vi "Set_up_measurement.vi"(4 "error in (no error)":errorcluster, 5 "VISA resource name":refnum<visa-resource-name>) -> (1 "error out":errorcluster, 2 "VISA resource name out":refnum<visa-resource-name>)   [LabVIEW 2021]
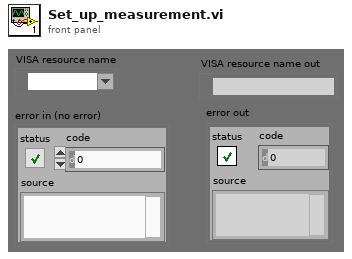
[diagram p1: front panel]
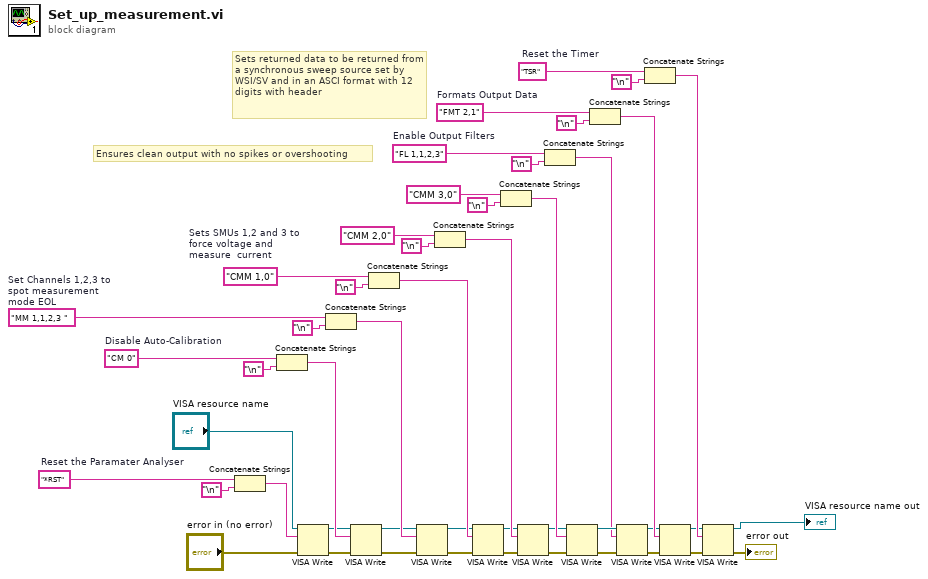
[diagram p0: block diagram]
diagram:
  w9 = "CM 0"  # Disable Auto-Calibration
  w12 = "*RST"  # Reset the Paramater Analyser
  w21 = "FMT 2,1"  # Formats Output Data
  w24 = "TSR"  # Reset the Timer
  w27 = "FL 1,1,2,3"  # Enable Output Filters
  w43 = "CMM 1,0"  # Sets SMUs 1,2 and 3 to force voltage and measure  current
  w47 = "MM 1,1,2,3 "  # Set Channels 1,2,3 to spot measurement mode EOL
  # "Sets returned data to be returned from a synchronous sweep source set by WSI/SV and in an ASCI format with 12 digits with header"
  # "Ensures clean output with no spikes or overshooting"
  n1 = Concatenate Strings(w12, "\n") -> (w10:string)
  n2 = Concatenate Strings(w9, "\n") -> (w7:string)
  n3 = VISA Write(VISA resource name="VISA resource name", write buffer=w10, error in (no error)="error in (no error)") -> (VISA resource name out=w6:refnum<visa-resource-name>, error out=w5:errorcluster)  [unwired: 1 out]
  n4 = Concatenate Strings(w47, "\n") -> (w45:string)
  n5 = VISA Write(VISA resource name=w6, write buffer=w7, error in (no error)=w5) -> (VISA resource name out=w2:refnum<visa-resource-name>, error out=w1:errorcluster)  [unwired: 1 out]
  n6 = Concatenate Strings(w43, "\n") -> (w44:string)
  n7 = VISA Write(VISA resource name=w2, write buffer=w45, error in (no error)=w1) -> (VISA resource name out=w41:refnum<visa-resource-name>, error out=w40:errorcluster)  [unwired: 1 out]
  n8 = Concatenate Strings("CMM 2,0" ("Sets SMUs 1,2 and 3 to force voltage and measure current"), "\n") -> (w39:string)
  n9 = VISA Write(VISA resource name=w41, write buffer=w44, error in (no error)=w40) -> (VISA resource name out=w35:refnum<visa-resource-name>, error out=w36:errorcluster)  [unwired: 1 out]
  n10 = Concatenate Strings("CMM 3,0" ("Sets SMUs 1,2 and 3 to force voltage and measure current"), "\n") -> (w34:string)
  n11 = VISA Write(VISA resource name=w35, write buffer=w39, error in (no error)=w36) -> (VISA resource name out=w31:refnum<visa-resource-name>, error out=w30:errorcluster)  [unwired: 1 out]
  n12 = Concatenate Strings(w27, "\n") -> (w25:string)
  n13 = VISA Write(VISA resource name=w31, write buffer=w34, error in (no error)=w30) -> (VISA resource name out=w28:refnum<visa-resource-name>, error out=w29:errorcluster)  [unwired: 1 out]
  n14 = Concatenate Strings(w21, "\n") -> (w19:string)
  n15 = VISA Write(VISA resource name=w28, write buffer=w25, error in (no error)=w29) -> (VISA resource name out=w18:refnum<visa-resource-name>, error out=w17:errorcluster)  [unwired: 1 out]
  n16 = Concatenate Strings(w24, "\n") -> (w22:string)
  n17 = VISA Write(VISA resource name=w18, write buffer=w19, error in (no error)=w17) -> (VISA resource name out=w16:refnum<visa-resource-name>, error out=w15:errorcluster)  [unwired: 1 out]
  n18 = VISA Write(VISA resource name=w16, write buffer=w22, error in (no error)=w15) -> (VISA resource name out=→"VISA resource name out":refnum<visa-resource-name>, error out=→"error out":errorcluster)  [unwired: 1 out]
